vi "Init.vi"(8 "error in (no error)":errorcluster, 10 "Settings":refnum<class "Progress Bar Settings.lvclass">, 11 "MGI_Progress Bar in":refnum<class "Progress Bar.lvclass">) -> (0 "error out":errorcluster, 3 "Progress Bar":refnum<data-value>)   [LabVIEW 2016, in "Progress Bar.lvclass"]
doc: "Call this VI before the loop to configure the look of the progress bar\n\nCopyright: MGI\nAuthored by: Derek Trepanier"
uses:
  <userlib>/_MGI/User Interface/Progress Bar/Progress Bar.lvclass
  <userlib>/_MGI/User Interface/Progress Bar/Progress Bar Settings/Progress Bar Settings.lvclass
  <userlib>/_MGI/User Interface/Progress Bar/Progress Bar.lvclass/Progress Bar.ctl
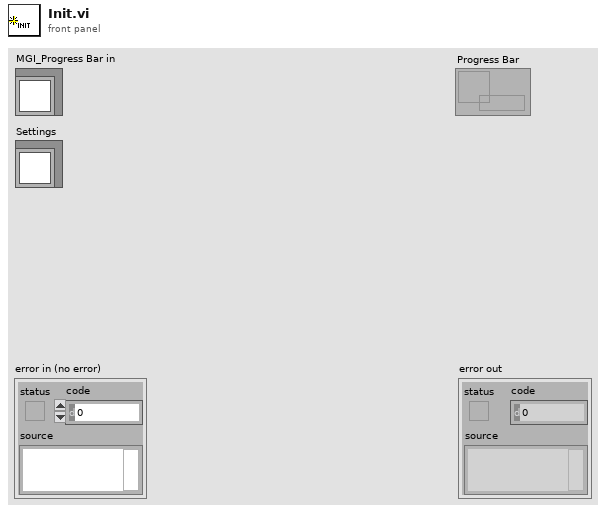
[diagram p1: front panel]
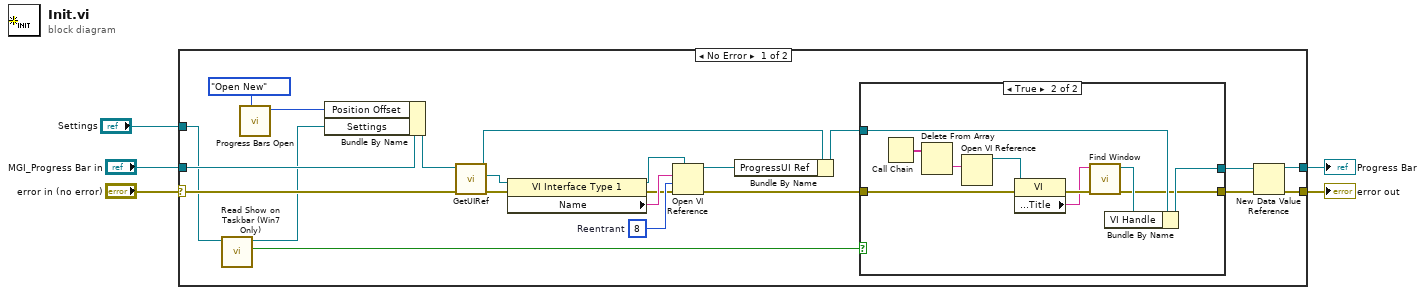
[diagram p0: block diagram]
diagram:
  n1 = case shown="No Error" "error in (no error)" {
    selector: "error in (no error)" -> [w22 w40]
    tunnel: [w26 w40] -> w4
    tunnel: "MGI_Progress Bar in" -> [w25 _]
    tunnel: [w27 _] -> w2
    tunnel: "Settings" -> [w14 _]
    frame No Error {
      w18 = 8  # Reentrant
      n2 = call-dynamic "Read Show on Taskbar (Win7 Only).vi"("MGI_Progress Bar Options in"=w14) -> ("Show on Taskbar (Win7 Only)"=w7:bool, "MGI_Progress Bar Options out"=w12:refnum<class "Progress Bar Settings.lvclass">)  [unwired: 8 in, 1 out]
      n3 = call <userlib>:"Progress Bars Open.vi"("Method"=enum16{"Open New", "Close", "Get"}."Open New") -> ("Open Progress Bars"=w13:i16)  [unwired: 10 in]
      n4 = Bundle By Name(cluster=w25, "Position Offset"=w13, "Settings"=w12) -> (w21:refnum<class "Progress Bar.lvclass">)
      n5 = call-dynamic "GetUIRef.vi"("error in (no error)"=w22, "MGI_Progress Bar in"=w21) -> ("error out"=w16:errorcluster, "VI Refnum"=w24:refnum<vi>, "MGI_Progress Bar out"=w23:refnum<class "Progress Bar.lvclass">)  [unwired: 7 in]
      n6 = property class="VI Interface Type 1"(reference=w24, error in=w16) -> (reference out=w20:refnum<vi>, error out=w15:errorcluster, "Name"=w19:string)
      n7 = Open VI Reference(type specifier VI Refnum (for type only)=w20, vi path=w19, options=w18, error in (no error)=w15) -> (vi reference=w6:refnum<vi>, error out=w8:errorcluster)  [unwired: 2 in]
      n8 = Bundle By Name(cluster=w23, "ProgressUI Ref"=w6) -> (w10:refnum<class "Progress Bar.lvclass">)
      n9 = case shown="True" w7 {
        tunnel: [w29 w38] -> w11
        tunnel: w10 -> [w29 w39]
        tunnel: [w28 w36] -> w9
        tunnel: w8 -> [w28 w35]
        frame False {
        }
        frame True {
          n10 = Call Chain() -> (call chain=w32:string[])
          n11 = Delete From Array(array=w32) -> (deleted portion=w31:string)  [unwired: 2 in, 1 out]
          n12 = Open VI Reference(vi path=w31) -> (vi reference=w30:refnum<vi>)  [unwired: 5 in, 1 out]
          n13 = property class="VI"(reference=w30, error in=w35) -> (error out=w34:errorcluster, "Front Panel.Title"=w33:string)  [unwired: 1 out]
          n14 = call <userlib>:"Find Window.vi"("error in (no error)"=w34, "Window Title (Callers Window)"=w33) -> ("error out"=w36:errorcluster, "Window Handle"=w37:refnum<k24>)  [unwired: 8 in]
          n15 = Bundle By Name(cluster=w39, "VI Handle"=w37) -> (w38:refnum<class "Progress Bar.lvclass">)
        }
      }
      n16 = New Data Value Reference(data value=w11, error in=w9) -> (data value reference=w27:refnum<data-value>, error out=w26:errorcluster)
    }
    frame Error {
    }
  }
  "error out" <- w4
  "Progress Bar" <- w2
